vi "Available Indicator Types.vi"() -> (2 "Element Types":map{string, refnum<class "GUI Element.lvclass">}(c390))   [LabVIEW 2020, in "VolatusGUI.lvlib"]
uses:
  VolatusGUI.lvlib
  GUI Element/GUI Element.lvclass
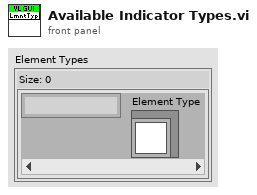
[diagram p1: front panel]
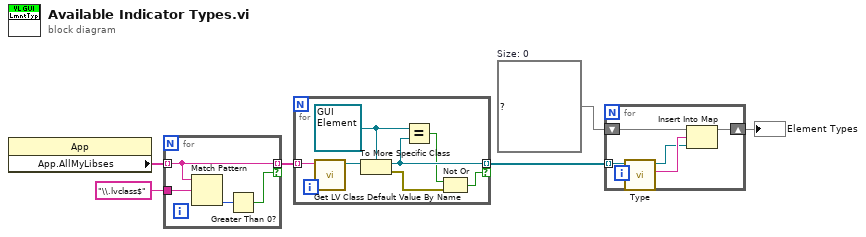
[diagram p0: block diagram]
diagram:
  w2 = map{string, refnum<class "GUI Element.lvclass">} {}  # Size: 0
  n1 = property class="App"() -> ("App.AllMyLibses"=w6:string[])  [unwired: 2 in, 2 out]
  n2 = for {
    tunnel: w6 -> [w10] mode=indexing
    tunnel: [w10] -> w4 mode=indexing if=w7
    tunnel: "\\.lvclass$" -> [w9]
    n3 = Match Pattern(string=w10, regular expression=w9) -> (offset past match=w8:i32)  [unwired: 1 in, 3 out]
    n4 = Greater Than 0?(x=w8) -> (x > 0?=w7:bool)
  }
  n5 = for {
    tunnel: w4 -> [w17] mode=indexing
    tunnel: [w15] -> w3 mode=indexing if=w11
    w14 = refnum<class "GUI Element.lvclass"> refnum ("VolatusGUI:GUI Element")
    n6 = call <vilib>:"Get LV Class Default Value By Name.vi"("class name"=w17) -> ("object"=w16:refnum<class>)  [unwired: 9 in, 1 out]
    n7 = To More Specific Class(target class=w14, reference=w16) -> (specific class reference=w15:refnum<class "GUI Element.lvclass">, error out=w13:errorcluster)  [unwired: 1 in]
    n8 = Equal?(x=w14, y=w15) -> (x = y?=w12:bool)
    n9 = Not Or(1:w13, 2:w12) -> (0:w11:bool)
  }
  n10 = for {
    tunnel: w3 -> [w19] mode=indexing
    shift-right: [w20] -> w1
    shift-left: w2 -> [w22]
    n11 = call "Type.vi"("GUI Element in"=w19) -> ("Element Type"=w21:string, "GUI Element out"=w18:refnum<class "GUI Element.lvclass">)  [unwired: 9 in]
    n12 = Insert Into Map(map in=w22, key=w21, value=w18) -> (map out=w20:map{string, refnum<class "GUI Element.lvclass">})  [unwired: 2 out]
  }
  "Element Types" <- w1
